vi "836_MultiCameraDirectly from IP Camera.vi"(7 "Operation":enum16{"Read", "Reopen", "Close"}(ring), 8 "error in":errorcluster, 9 "Camera Settings":T2={"fps"=30, "compression"=30, "Image Size"=enum."320x240"}, 10 "Image":T1, 11 "address":string="10.te.am.11") -> (0 "error out":errorcluster, 1 "Bandwidth (Mbps)":dbl=30.0, 2 "Image Out":T1)   [LabVIEW 2015]
doc: "This VI is intended for testing, examples, and demos. It assumes the camera is directly accssible from the computer and not the robot. It retrieves an image from either a USB or IP Axis camera.\n\nThis software is licensed. Open the labview\\readme\\WPI Robotics Library Open Source License.txt file for more information."
uses:
  <vilib>/Rock Robotics/WPI/Camera/WPI_CameraSettings Read MJPG.ctl
  <vilib>/Rock Robotics/WPI/Camera/WPI_CameraImageSize.ctl
  <vilib>/vision/Image Controls.llb/IMAQ Image.ctl
  <vilib>/picture/picture.llb/imagedata.ctl
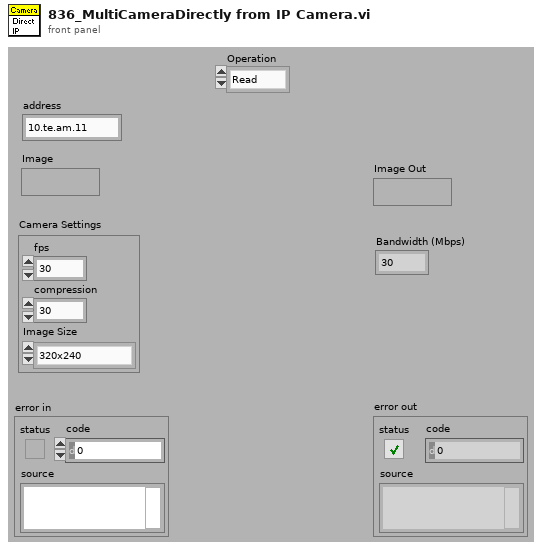
[diagram p1: front panel]
types:
  T1 = typedef "IMAQ Image.ctl" = refnum<image>
  T2 = typedef "WPI_CameraSettings Read MJPG.ctl" = cluster{"fps":i32, "compression":i32, "Image Size":T3}
  T3 = typedef "WPI_CameraImageSize.ctl" = enum16{"640x480", "320x240", "160x120", "Custom"}
  T4 = typedef "imagedata.ctl" = cluster{"image type":i32, "image depth":i32, "image":u8[], "mask":u8[], "colors":u32[], "Rectangle":cluster{"left":i16, "top":i16, "right":i16, "bottom":i16}}
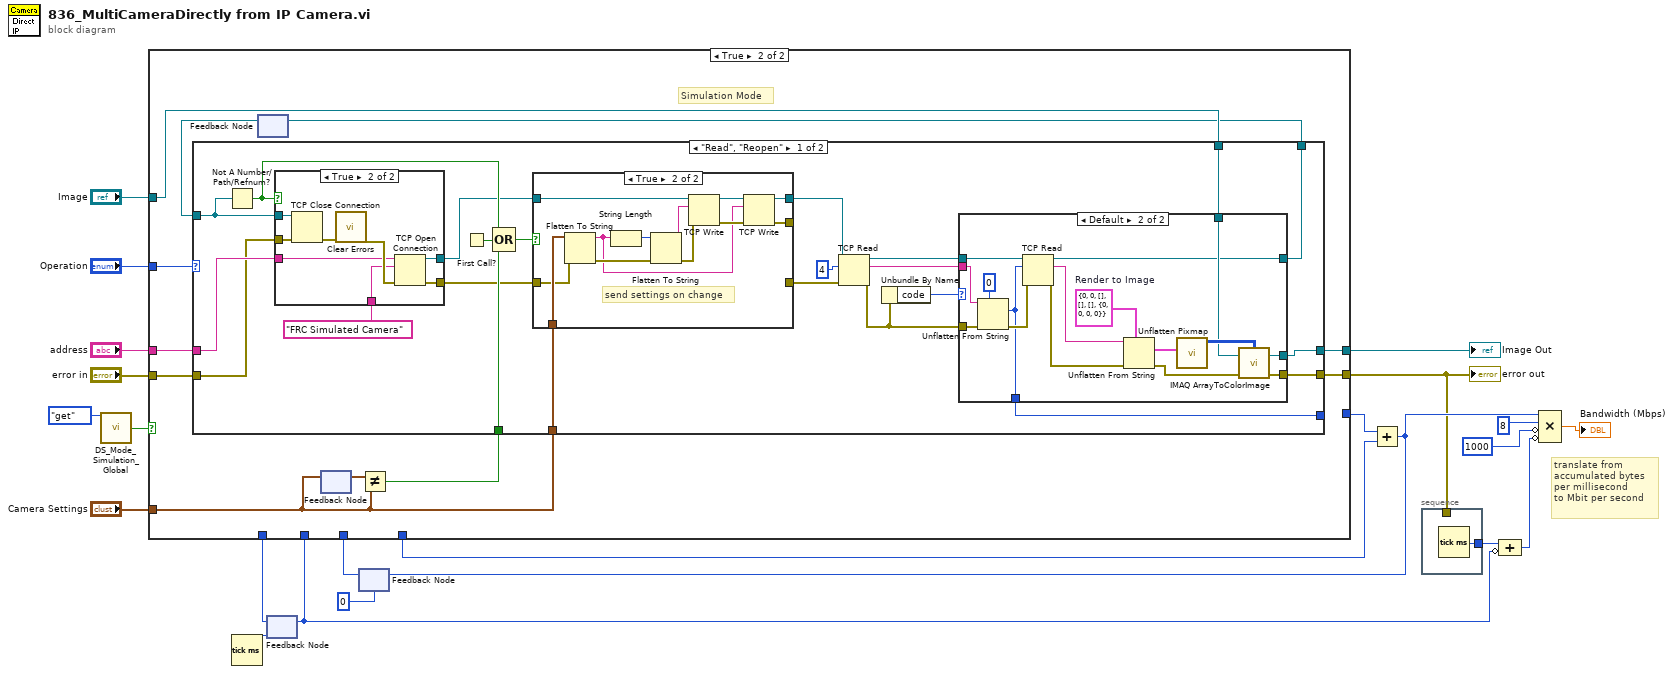
[diagram p0: block diagram]
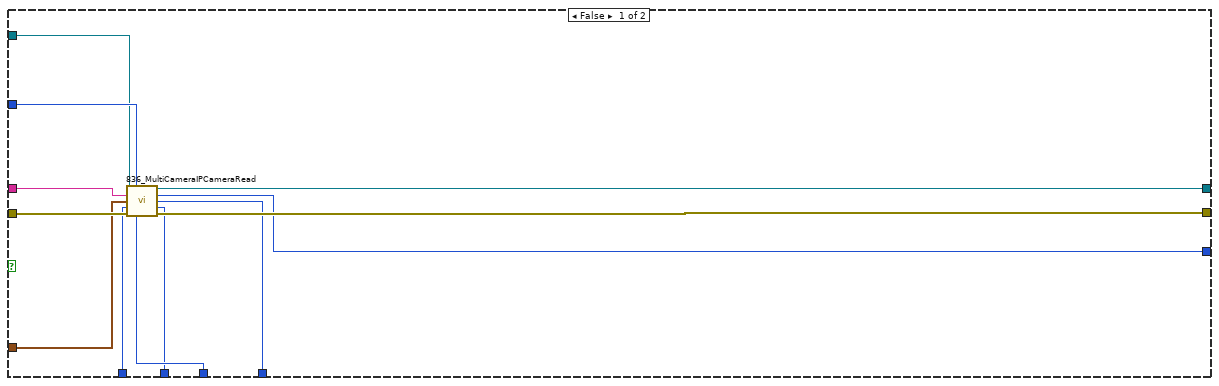
[diagram p2: hidden frame]
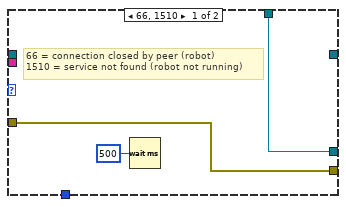
[diagram p4: hidden frame]
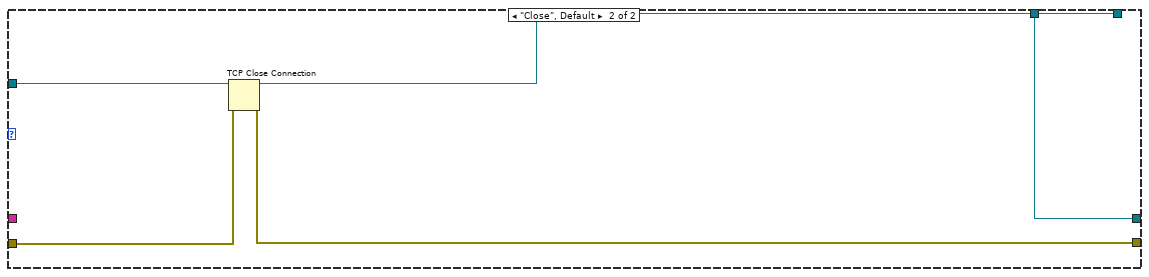
[diagram p6: hidden frame]
diagram:
  # "translate from\naccumulated bytes\nper millisecond \nto Mbit per second"
  n1 = call <vilib>:"DS_Mode_Simulation_Global.vi"("menu"=enum16{"set", "get"}."get") -> ("simulated? out"=w17:bool)  [unwired: 13 in, 1 out]
  n2 = Tick Count (ms)() -> (millisecond timer value=w14:u32)
  n3 = feedback #1(w14) -> (w9:u32)
  n4 = feedback #2(0) -> (w11:i32)
  n5 = case shown="True" w17 {
    tunnel: "error in" -> [w34 w43]
    tunnel: "address" -> [w23 w44]
    tunnel: [w33 w42] -> w20
    tunnel: [w32 w41] -> w4
    tunnel: "Operation" -> [w31 w39]
    tunnel: "Image" -> [w30 w40]
    tunnel: [w29 _] -> w7
    tunnel: w11 -> [w28 _]
    tunnel: [w27 _] -> w10
    tunnel: w9 -> [w26 _]
    tunnel: [w25 _] -> w5
    tunnel: "Camera Settings" -> [w24 w36]
    frame False {
      n6 = call "836_MultiCameraIPCameraRead.vi"("Refnum in"=w30, "Operation"=w31, "address"=w23, "Camera Settings"=w24, "millisecond timer value in"=w26, "error in (no error)"=w34, "Numeric in"=w28) -> ("Refnum out"=w33:T1, "Numeric 3"=w29:i32, "Numeric out"=w27:i32, "millisecond timer value out"=w25:u32, "error out"=w32:errorcluster)  [unwired: 4 in]
    }
    frame True {
      # "Simulation Mode"
      n7 = feedback #3() -> (w45:refnum<k5>)  [unwired: 1 out]
      n8 = feedback-in #4(w36) -> ()
      n9 = feedback #4() -> (w37:T2)  [unwired: 1 in]
      n10 = Not Equal?(x=w37, y=w36) -> (x != y?=w35:bool)
      n11 = case shown="\"Read\", \"Reopen\"" w39 {
        tunnel: w45 -> [w68 w116]
        tunnel: w44 -> [w67 _]
        tunnel: w43 -> [w66 w115]
        tunnel: [w65 w113] -> w42
        tunnel: [w56 w114] -> w41
        tunnel: w40 -> [w64 w113]
        tunnel: [w58 _] -> _
        tunnel: w36 -> [w49 _]
        tunnel: [w57 w112] -> w38
        tunnel: w35 -> [w53 _]
        frame "Read", "Reopen" {
          n12 = Not A Number/Path/Refnum?(number/path/refnum=w68) -> (NaN/Path/Refnum?=w52:bool)
          n13 = case shown="True" w52 {
            tunnel: w68 -> [w103 w111]
            tunnel: w67 -> [_ w105]
            tunnel: [w103 w108] -> w51
            tunnel: w66 -> [w102 w107]
            tunnel: [w102 w106] -> w48
            tunnel: "FRC Simulated Camera" ("service name") -> [_ w104]
            frame False {
            }
            frame True {
              n14 = TCP Close Connection(connection ID=w111, error in (no error)=w107) -> (error out=w110:errorcluster)  [unwired: 2 out]
              n15 = call <vilib>:"Clear Errors.vi"("error in (no error)"=w110) -> ("error out"=w109:errorcluster)  [unwired: 1 in, 5 out]
              n16 = TCP Open Connection(address=w105, remote port or service name=w104, error in (no error)=w109) -> (connection ID=w108:refnum<k5>, error out=w106:errorcluster)  [unwired: 2 in]
            }
          }
          n17 = First Call?() -> (First Call?: T/F=w55:bool)
          n18 = Compound Arithmetic op=OR(w52, w55, w53) -> (w54:bool)
          n19 = case shown="True" w54 {
            tunnel: w51 -> [w70 w82]
            tunnel: w49 -> [_ w80]
            tunnel: [w70 w73] -> w50
            tunnel: w48 -> [w69 w72]
            tunnel: [w69 _] -> w47
            tunnel: [_ w71] -> _
            frame False {
            }
            frame True {
              # "send settings on change"
              n20 = Flatten To String(anything=w80, error in (no error)=w72) -> (data string=w74:string, error out=w76:errorcluster)  [unwired: 2 in, 1 out]
              n21 = String Length(string=w74) -> (length=w81:i32)
              n22 = Flatten To String(anything=w81, error in (no error)=w76) -> (data string=w79:string, error out=w77:errorcluster)  [unwired: 2 in, 1 out]
              n23 = TCP Write(connection ID=w82, data in=w79, error in (no error)=w77) -> (connection ID out=w75:refnum<k5>, error out=w78:errorcluster)  [unwired: 1 in, 1 out]
              n24 = TCP Write(connection ID=w75, data in=w74, error in (no error)=w78) -> (connection ID out=w73:refnum<k5>, error out=w71:errorcluster)  [unwired: 1 in, 1 out]
            }
          }
          n25 = TCP Read(connection ID=w50, bytes to read=4, error in (no error)=w47) -> (connection ID out=w61:refnum<k5>, data out=w62:string, error out=w60:errorcluster)  [unwired: 1 in, 1 out]
          n26 = Unbundle By Name(w60) -> ("code"=w59:i32)
          n27 = case shown="Default" w59 {
            tunnel: [w85 w97] -> w65
            tunnel: [w84 w86] -> w56
            tunnel: w64 -> [w85 w96]
            tunnel: w62 -> [_ w95]
            tunnel: w61 -> [_ w94]
            tunnel: w60 -> [w84 w92]
            tunnel: [_ w90] -> w58
            tunnel: [_ w87] -> w57
            frame 66, 1510 {
              # "66 = connection closed by peer (robot)\n1510 = service not found (robot not running)"
              n28 = Wait (ms)(milliseconds to wait=u32 500) -> ()  [unwired: 1 out]
            }
            frame Default {
              w99 = T4 {"image type"=0, "image depth"=0, "image"=[], "mask"=[], "colors"=[], "Rectangle"={"left"=0, "top"=0, "right"=0, "bottom"=0}}  # Render to Image
              n29 = Unflatten From String(type=0 ("bytes to read"), binary string=w95, error in (no error)=w92) -> (value=w90:i32, error out=w91:errorcluster)  [unwired: 2 in, 1 out]
              n30 = TCP Read(connection ID=w94, bytes to read=w90, error in (no error)=w91) -> (connection ID out=w87:refnum<k5>, data out=w98:string, error out=w89:errorcluster)  [unwired: 1 in, 1 out]
              n31 = Unflatten From String(type=w99, binary string=w98, error in (no error)=w89) -> (value=w100:T4, error out=w88:errorcluster)  [unwired: 2 in, 1 out]
              n32 = call <vilib>:"Unflatten Pixmap.vi"("image data"=w100) -> ("24-bit pixmap"=w101:u32[][])  [unwired: 4 in, 6 out]
              n33 = call "IMAQ ArrayToColorImage"("Image Pixels (U32)"=w101, "Image"=w96, "error in (no error)"=w88) -> ("Image Out"=w97:T1, "error out"=w86:errorcluster)  [unwired: 2 in]
            }
          }
        }
        frame "Close", Default {
          n34 = TCP Close Connection(connection ID=w116, error in (no error)=w115) -> (connection ID out=w112:refnum<k5>, error out=w114:errorcluster)  [unwired: 1 out]
        }
      }
      n35 = feedback-in #3(w38) -> ()
    }
  }
  "Image Out" <- w20
  "error out" <- w4
  n36 = feedback-in #1(w5) -> ()
  n37 = Add(x=w7, y=w10) -> (x+y=w8:i32)
  n38 = feedback-in #2(w8) -> ()
  n39 = stacked-sequence {
    tunnel: [w117] -> w6
    tunnel: w4 -> [_]
    frame #0 {
      n40 = Tick Count (ms)() -> (millisecond timer value=w117:u32)
    }
  }
  n41 = Compound Arithmetic op=ADD(w6, invert w5) -> (w3:u32)
  n42 = Compound Arithmetic op=MULTIPLY(w8, 8 ("timeout ms (25000)"), invert 1000 ("timeout ms (25000)"), invert w3) -> (→"Bandwidth (Mbps)":dbl)
